vi "Nested Core.vi"(8 "error in (no error)":errorcluster, 10 "key":string, 11 "JSON Datatype in":refnum<class "JSON Datatype.lvclass">) -> (0 "error out":errorcluster, 1 "found":bool, 2 "stop?":bool, 3 "JSON Datatype out":refnum<class "JSON Datatype.lvclass">)   [LabVIEW 2015, in "LVJSON.lvlib" / "JSON Object.lvclass"]
uses:
  JSON Object.lvclass
  JSON Datatype/JSON Datatype.lvclass
  JSON Datatype/To More Specific Type (Object).vi
  Get Value (JSON).vi
  JSON Datatype/To More Specific Type (Array).vi
  JSON Array/Index Array (JSON).vi
  JSON Array/JSON Array.lvclass
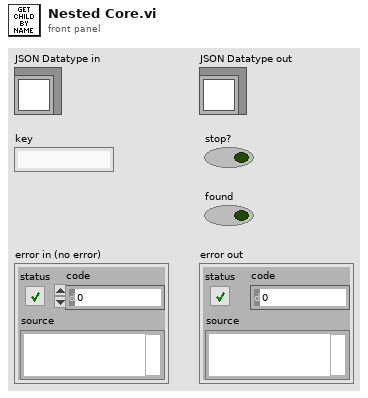
[diagram p1: front panel]
types:
  T1 = typedef "LVJSON.lvlib/JSON Types.ctl" = enum16{"String", "Numeric", "Boolean", "NULL", "Object", "Array", "Unknown"}
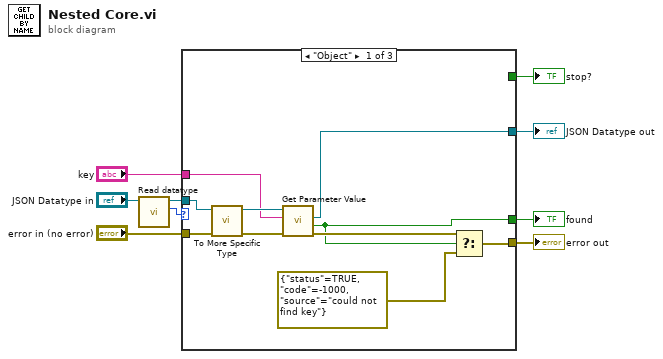
[diagram p0: block diagram]
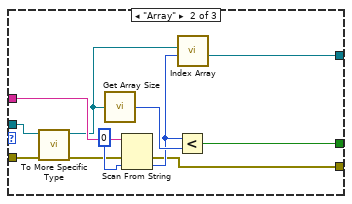
[diagram p2: hidden frame]
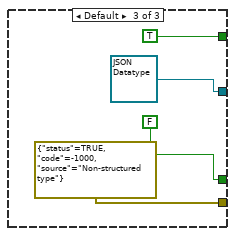
[diagram p3: hidden frame]
diagram:
  n1 = call-dynamic "Read datatype.vi"("JSON Datatype in"="JSON Datatype in") -> ("datatype"=w2:T1, "JSON Datatype out"=w1:refnum<class "JSON Datatype.lvclass">)  [unwired: 8 in, 1 out]
  n2 = case shown="\"Object\"" w2 {
    tunnel: "key" -> [w12 w29 _]
    tunnel: [w10 w27 refnum<class "JSON Datatype.lvclass"> refnum ("JSON Data")] -> w9
    tunnel: w1 -> [w19 w30 _]
    tunnel: [w15 w21 errorcluster {"status"=TRUE, "code"=-1000, "source"="Non-structured type"} ("f")] -> w5
    tunnel: "error in (no error)" -> [w18 w26 _]
    tunnel: [_ _ TRUE] -> w7
    tunnel: [w11 w20 FALSE] -> w8
    frame "Object" {
      n3 = call-poly "To More Specific Type.vi"("error in (no error)"=w18, "JSON Datatype in"=w19) -> ("error out"=w17:errorcluster, "JSON Datatype out"=w13:refnum<class "JSON Object.lvclass">)  [unwired: 8 in]
      n4 = call-poly "Get Parameter Value.vi"("error in (no error)"=w17, "key"=w12, "JSON Object in"=w13) -> ("error out"=w16:errorcluster, "found"=w11:bool, "value"=w10:refnum<class "JSON Datatype.lvclass">)  [unwired: 6 in]
      n5 = Select(t=w16, s=w11, f=errorcluster {"status"=TRUE, "code"=-1000, "source"="could not find key"}) -> (s? t:f=w15:errorcluster)
    }
    frame "Array" {
      n6 = call-poly "To More Specific Type.vi"("error in (no error)"=w26, "JSON Datatype in"=w30) -> ("error out"=w25:errorcluster, "JSON Datatype out"=w24:refnum<class "JSON Array.lvclass">)  [unwired: 8 in]
      n7 = call "Get Array Size.vi"("JSON Array in"=w24) -> ("size(s)"=w23:i32)
      n8 = Scan From String(input string=w29, error in=w25, default 1=0 ("index")) -> (error out=w21:errorcluster, output 1=w22:i32)  [unwired: 2 in, 2 out]
      n9 = Less?(x=w22, y=w23) -> (x < y?=w20:bool)
      n10 = call-poly "Index Array.vi"("index"=w22, "JSON Array in"=w24) -> ("JSON Data"=w27:refnum<class "JSON Datatype.lvclass">)  [unwired: 9 in]
    }
    frame Default {
    }
  }
  "JSON Datatype out" <- w9
  "found" <- w8
  "stop?" <- w7
  "error out" <- w5
